vi "Actor Core.vi"(8 "error in":errorcluster, 11 "Room Service Manager UI in":refnum<class "Room Service Manager UI.lvclass">) -> (0 "error out":errorcluster, 3 "Actor out":refnum<class "Actor.lvclass">)   [LabVIEW 2023, in "Room Service Manager UI.lvlib" / "Room Service Manager UI.lvclass"]
doc: "(<B>Filename</B>: Actor Framework.lvlib:Actor.lvclass:Actor Core.vi)\n\nReceives messages to the actor, reacts to them, and initiates any error handling that may shut the actor down.\n\nDescendant classes may override this VI to append parallel tasks for the actor to complete while it handles messages. Overrides use the Call Parent Class Method node."
uses:
  Room Service Manager UI.lvclass
  Room Service Manager UI.lvclass/Room Service Manager UI.ctl
  <vilib>/ActorFramework/Stop Msg/Stop Msg.lvclass
  <vilib>/ActorFramework/Actor/Actor.lvclass
  C:/Users/bhaghyaraj/Trainings/NI Actor Framework/SDLC/UI Base/UI Base/UI Base.lvclass
  C:/Program Files/National Instruments/LabVIEW 2023/vi.lib/ActorFramework/Actor/Actor.lvclass
  C:/Users/bhaghyaraj/Trainings/NI Actor Framework/SDLC/Room Service Manager UI/Room Service Manager UI/Room Service Manager UI.lvclass
  UI Base/UI Base/UI Base.lvclass
panel:
  in  "Service State":T1(tab)
  in  "Other Request":bool
  in  "Food Order":bool
  in  "HouseKeeping":bool
  in  "Room Cleaning":bool
  in  "Laundry":bool
  in  "Request":bool
  in  "Request Details":string
  in  "Other Request 2":bool
  out "Title":string
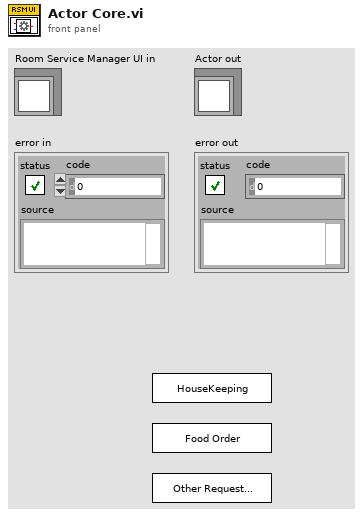
[diagram p1: front panel]
types:
  T1 = enum32{"Home", "HouseKeeping", "Food Order", "Other Request"}
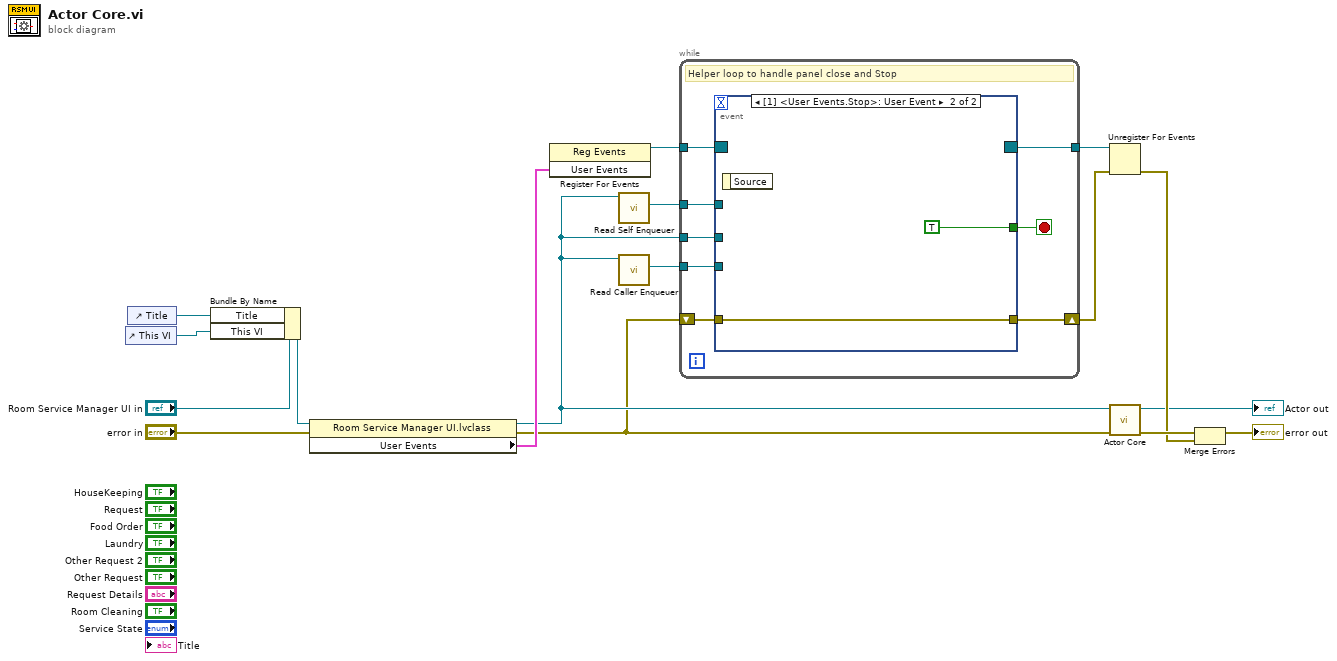
[diagram p0: block diagram]
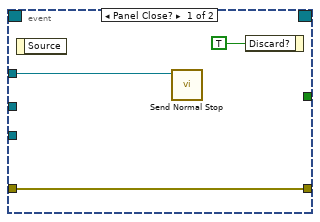
[diagram p2: hidden frame]
diagram:
  n1 = control-ref of="This VI"() -> (w1:refnum<vi>)
  n2 = control-ref of="Title"() -> (w2:refnum<vi>)
  n3 = Bundle By Name(cluster="Room Service Manager UI in", "Title"=w2, "This VI"=w1) -> (w3:refnum<class "Room Service Manager UI.lvclass">)
  n4 = property class="Room Service Manager UI.lvclass"(reference=w3, error in="error in") -> (reference out=w10:refnum<class "Room Service Manager UI.lvclass">, error out=w9:errorcluster, "User Events"=w13:cluster{"Stop":refnum<user-event>})
  n5 = register-events(w13) -> (reference out=w15:refnum<event-registration>)  [unwired: 2 in, 1 out]
  n6 = call <vilib>:"Read Self Enqueuer.vi"("Actor"=w10) -> ("Self Enqueuer"=w14:refnum<class "Message Enqueuer.lvclass">)  [unwired: 10 in]
  n7 = call <vilib>:"Read Caller Enqueuer.vi"("Actor"=w10) -> ("Caller Enqueuer"=w11:refnum<class "Message Enqueuer.lvclass">)  [unwired: 10 in]
  n8 = while {
    tunnel: w14 -> [w25]
    tunnel: w15 -> [w24]
    tunnel: [w22] -> w16
    tunnel: w11 -> [w21]
    tunnel: w10 -> [w20]
    shift-right: [w18] -> w8
    shift-left: w9 -> [w19]
    stop <- w23 stop-if-true
    # "Helper loop to handle panel close and Stop"
    n9 = event shown="[1] <User Events.Stop>: User Event" {
      selector: w24 -> [_ _]
      dyn-events: [_ _] -> w22
      timeout: _ -> [_ _]
      tunnel: w25 -> [w27 _]
      tunnel: [_ TRUE] -> w23
      tunnel: w21 -> [_ _]
      tunnel: w20 -> [_ _]
      tunnel: w19 -> [w26 w29]
      tunnel: [w26 w29] -> w18
      event Panel Close? {
        n10 = event-data() -> ()  [unwired: 1 in, 1 out]
        n11 = call <vilib>:"Send Normal Stop.vi"("Message Enqueuer"=w27) -> ()  [unwired: 10 in, 1 out]
        n12 = event-data("Discard?"=TRUE) -> ()  [unwired: 1 in, 1 out]
      }
      event User Event {
        n13 = event-data() -> ()  [unwired: 1 in, 1 out]
      }
    }
  }
  n14 = Unregister For Events(event registration refnum=w16, error in=w8) -> (error out=w12:errorcluster)
  n15 = call-parent "Actor Core.vi"("error in"=w9, "Actor in"=w10) -> ("error out"=w17:errorcluster, "Actor out"=→"Actor out":refnum<class "Actor.lvclass">)  [unwired: 8 in]
  n16 = Merge Errors(w17, w12) -> (→"error out":errorcluster)
